vi "read_esp32_Hall_value.vi"() -> ()   [LabVIEW 2021]
uses:
  <vilib>/Instr/_visa.llb/VISA Configure Serial Port (Instr).vi
panel:
  out "Waveform Chart":i32(graph)
  in  "byte count":u32
  out "ÀNº¸­È":string
  in  "com port":refnum<visa-resource-name>
  in  "stop":bool
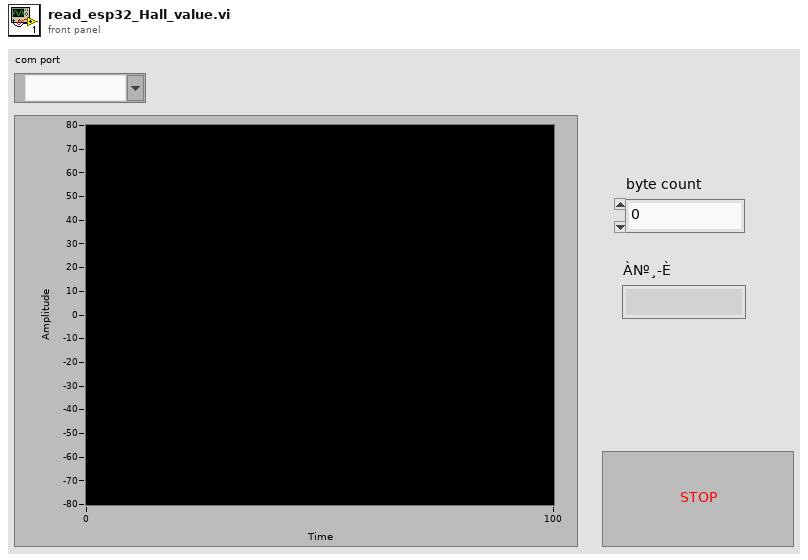
[diagram p1: front panel]
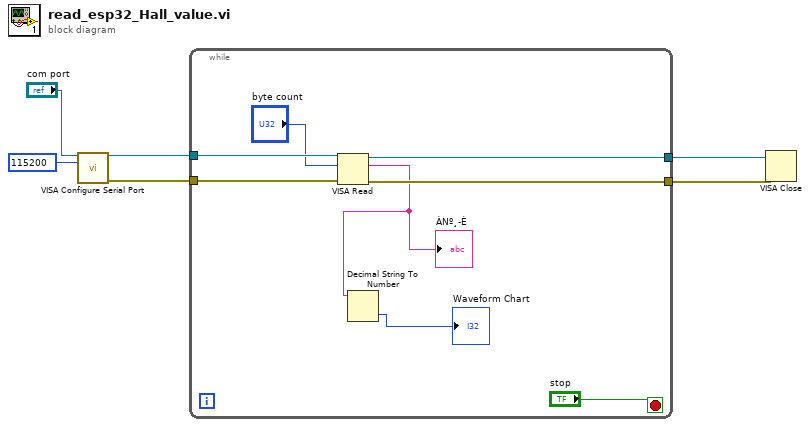
[diagram p0: block diagram]
diagram:
  n1 = call-poly "VISA Configure Serial Port"("VISA resource name"="com port", "baud rate (9600)"=u32 115200) -> ("VISA resource name out"=w4:refnum<visa-resource-name>, "error out"=w3:errorcluster)  [unwired: 12 in]
  n2 = while {
    tunnel: w4 -> [w13]
    tunnel: w3 -> [w12]
    tunnel: [w11] -> w2
    tunnel: [w10] -> w1
    stop <- "stop" stop-if-true
    n3 = VISA Read(VISA resource name=w13, byte count="byte count", error in (no error)=w12) -> (VISA resource name out=w10:refnum<visa-resource-name>, read buffer=w8:string, error out=w11:errorcluster)  [unwired: 1 out]
    "ÀNº¸­È" <- w8
    n4 = Decimal String To Number(string=w8) -> (number=→"Waveform Chart":i32)  [unwired: 2 in, 1 out]
  }
  n5 = VISA Close(VISA resource name=w1, error in (no error)=w2) -> ()  [unwired: 1 out]
